vi "ParseSlaveRWw.vi"(1 "Node RWw":u16[][](array[numeric])) -> (0 "力觉力":sgl[](array[numeric]) format="%.2f")   [LabVIEW 2018]
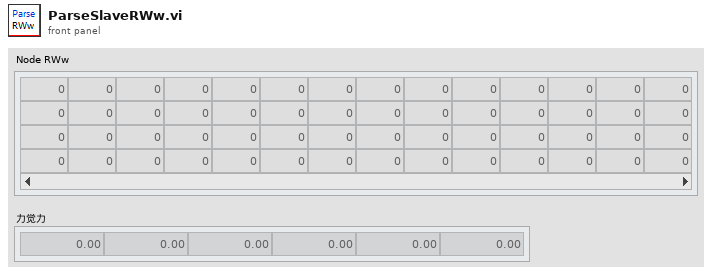
[diagram p1: front panel]
types:
  T1 = cluster{"1#当前泄漏量":sgl, "1#稳定泄漏量":sgl, "1#当前压力":sgl, "1#稳定压力":sgl, "1#风门闭电压":sgl, "1#风门开电压":sgl, "1#LED电流":sgl, "1#LED电压":sgl, "2#当前泄漏量":sgl, "2#稳定泄漏量":sgl, "2#当前压力":sgl, "2#稳定压力":sgl, "2#风门闭电压":sgl, "2#风门开电压":sgl, "2#LED电流":sgl, "2#LED电压":sgl, "3#当前泄漏量":sgl, "3#稳定泄漏量":sgl, "3#当前压力":sgl, "3#稳定压力":sgl, "3#风门闭电压":sgl, "3#风门开电压":sgl, "3#LED电流":sgl, "3#LED电压":sgl}
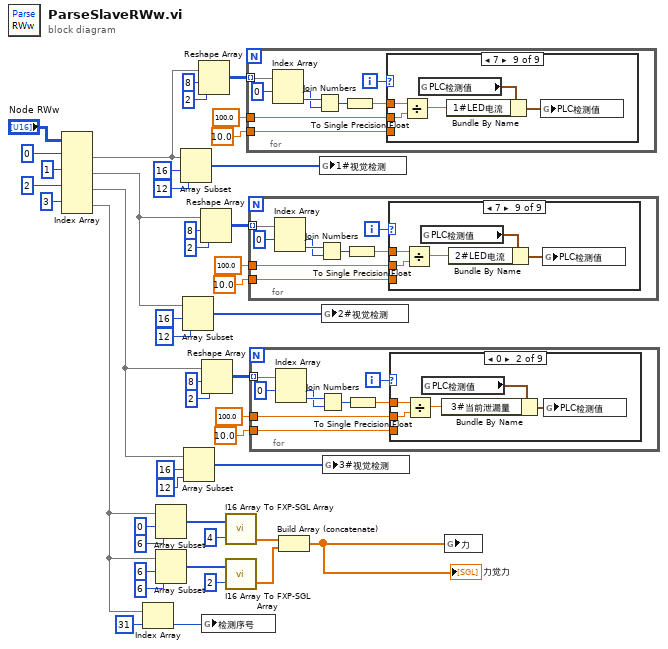
[diagram p0: block diagram]
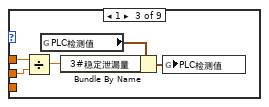
[diagram p3: hidden frame]
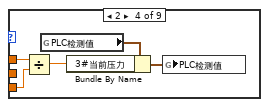
[diagram p4: hidden frame]
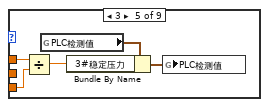
[diagram p5: hidden frame]
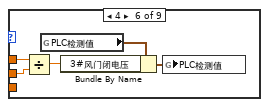
[diagram p6: hidden frame]
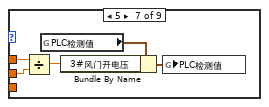
[diagram p7: hidden frame]
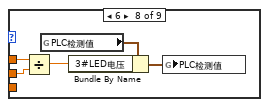
[diagram p8: hidden frame]
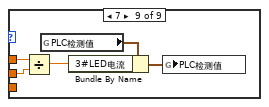
[diagram p9: hidden frame]
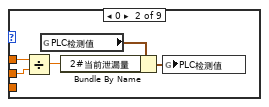
[diagram p11: hidden frame]
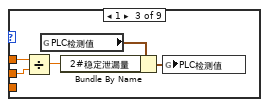
[diagram p12: hidden frame]
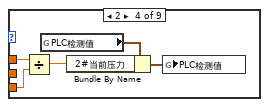
[diagram p13: hidden frame]
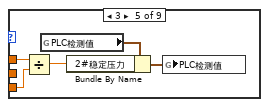
[diagram p14: hidden frame]
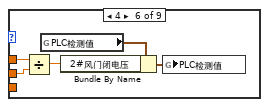
[diagram p15: hidden frame]
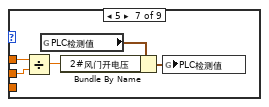
[diagram p16: hidden frame]
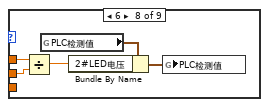
[diagram p17: hidden frame]
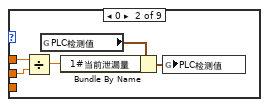
[diagram p19: hidden frame]
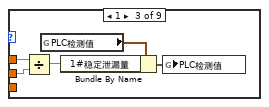
[diagram p20: hidden frame]
diagram:
  n1 = Index Array(array="Node RWw", index (row) #1=0 ("索引 (行)"), index (row) #2=1 ("索引 (行)"), index (row) #3=2 ("索引 (行)"), index (row) #4=3 ("索引 (行)")) -> (element #1=w39:u16[], element #2=w15:u16[], element #3=w6:u16[], element #4=w3:u16[])  [unwired: 4 in]
  n2 = Index Array(array=w3, index=31 ("索引")) -> (element=w1:u16)
  n3 = Array Subset(array=w3, index=0 ("索引"), length=6 ("长度")) -> (w33:u16[])
  n4 = Array Subset(array=w3, index=6 ("索引"), length=6 ("长度")) -> (w28:u16[])
  n5 = Array Subset(array=w39, index=16 ("索引"), length=12 ("长度")) -> (w36:u16[])
  n6 = Array Subset(array=w15, index=16 ("索引"), length=12 ("长度")) -> (w16:u16[])
  n7 = Array Subset(array=w6, index=16 ("索引"), length=12 ("长度")) -> (w7:u16[])
  n8 = Reshape Array(w39, 8 ("维数大小"), 2 ("维数大小")) -> (w42:u16[][])
  n9 = Reshape Array(w15, 8 ("维数大小"), 2 ("维数大小")) -> (w21:u16[][])
  n10 = Reshape Array(w6, 8 ("维数大小"), 2 ("维数大小")) -> (w12:u16[][])
  n11 = global write "全局 1.vi" "检测序号"(w1) -> ()
  n12 = call "I16 Array To FXP-SGL Array.vi"("小数位数"=4, "I16 Array"=w33) -> ("SGL Array"=w26:sgl[])  [unwired: 1 out]
  n13 = call "I16 Array To FXP-SGL Array.vi"("小数位数"=2, "I16 Array"=w28) -> ("SGL Array"=w25:sgl[])  [unwired: 1 out]
  n14 = for {
    tunnel: w42 -> [w55] mode=indexing
    tunnel: sgl 100.0 -> [w49]
    tunnel: sgl 10.0 -> [w48]
    i -> [w47]
    n15 = Index Array(array=w55, index #1=0 ("索引")) -> (element #1=w52:u16, element #2=w53:u16)  [unwired: 1 in]
    n16 = Join Numbers(hi=w53, lo=w52) -> ((hi.lo)=w51:u32)
    n17 = To Single Precision Float(number=w51) -> (single precision float=w50:sgl)
    n18 = case shown="7" w47 {
      tunnel: w50 -> [_ w60 w65 w70 w75 w80 w85 w90 w95]
      tunnel: w49 -> [_ w59 w64 _ _ w79 w84 w89 w91]
      tunnel: w48 -> [_ _ _ w66 w71 _ _ _ _]
      frame -1, Default {
      }
      frame 0 {
        n19 = Divide(x=w60, y=w59) -> (x/y=w58:sgl)
        n20 = global read "全局 1.vi" "PLC检测值"() -> (w56:T1)
        n21 = Bundle By Name(cluster=w56, "1#当前泄漏量"=w58) -> (w57:T1)
        n22 = global write "全局 1.vi" "PLC检测值"(w57) -> ()
      }
      frame 1 {
        n23 = Divide(x=w65, y=w64) -> (x/y=w63:sgl)
        n24 = global read "全局 1.vi" "PLC检测值"() -> (w61:T1)
        n25 = Bundle By Name(cluster=w61, "1#稳定泄漏量"=w63) -> (w62:T1)
        n26 = global write "全局 1.vi" "PLC检测值"(w62) -> ()
      }
      frame 2 {
        n27 = Divide(x=w70, y=w66) -> (x/y=w69:sgl)
        n28 = global read "全局 1.vi" "PLC检测值"() -> (w67:T1)
        n29 = Bundle By Name(cluster=w67, "1#当前压力"=w69) -> (w68:T1)
        n30 = global write "全局 1.vi" "PLC检测值"(w68) -> ()
      }
      frame 3 {
        n31 = Divide(x=w75, y=w71) -> (x/y=w74:sgl)
        n32 = global read "全局 1.vi" "PLC检测值"() -> (w72:T1)
        n33 = Bundle By Name(cluster=w72, "1#稳定压力"=w74) -> (w73:T1)
        n34 = global write "全局 1.vi" "PLC检测值"(w73) -> ()
      }
      frame 4 {
        n35 = Divide(x=w80, y=w79) -> (x/y=w78:sgl)
        n36 = global read "全局 1.vi" "PLC检测值"() -> (w76:T1)
        n37 = Bundle By Name(cluster=w76, "1#风门闭电压"=w78) -> (w77:T1)
        n38 = global write "全局 1.vi" "PLC检测值"(w77) -> ()
      }
      frame 5 {
        n39 = Divide(x=w85, y=w84) -> (x/y=w83:sgl)
        n40 = global read "全局 1.vi" "PLC检测值"() -> (w81:T1)
        n41 = Bundle By Name(cluster=w81, "1#风门开电压"=w83) -> (w82:T1)
        n42 = global write "全局 1.vi" "PLC检测值"(w82) -> ()
      }
      frame 6 {
        n43 = Divide(x=w90, y=w89) -> (x/y=w88:sgl)
        n44 = global read "全局 1.vi" "PLC检测值"() -> (w86:T1)
        n45 = Bundle By Name(cluster=w86, "1#LED电压"=w88) -> (w87:T1)
        n46 = global write "全局 1.vi" "PLC检测值"(w87) -> ()
      }
      frame 7 {
        n47 = Divide(x=w95, y=w91) -> (x/y=w94:sgl)
        n48 = global read "全局 1.vi" "PLC检测值"() -> (w92:T1)
        n49 = Bundle By Name(cluster=w92, "1#LED电流"=w94) -> (w93:T1)
        n50 = global write "全局 1.vi" "PLC检测值"(w93) -> ()
      }
    }
  }
  n51 = for {
    tunnel: w21 -> [w104] mode=indexing
    tunnel: sgl 100.0 -> [w98]
    tunnel: sgl 10.0 -> [w97]
    i -> [w96]
    n52 = Index Array(array=w104, index #1=0 ("索引")) -> (element #1=w101:u16, element #2=w102:u16)  [unwired: 1 in]
    n53 = Join Numbers(hi=w102, lo=w101) -> ((hi.lo)=w100:u32)
    n54 = To Single Precision Float(number=w100) -> (single precision float=w99:sgl)
    n55 = case shown="7" w96 {
      tunnel: w99 -> [_ w109 w114 w119 w124 w129 w134 w139 w144]
      tunnel: w98 -> [_ w108 w113 _ _ w128 w133 w138 w140]
      tunnel: w97 -> [_ _ _ w115 w120 _ _ _ _]
      frame -1, Default {
      }
      frame 0 {
        n56 = Divide(x=w109, y=w108) -> (x/y=w107:sgl)
        n57 = global read "全局 1.vi" "PLC检测值"() -> (w105:T1)
        n58 = Bundle By Name(cluster=w105, "2#当前泄漏量"=w107) -> (w106:T1)
        n59 = global write "全局 1.vi" "PLC检测值"(w106) -> ()
      }
      frame 1 {
        n60 = Divide(x=w114, y=w113) -> (x/y=w112:sgl)
        n61 = global read "全局 1.vi" "PLC检测值"() -> (w110:T1)
        n62 = Bundle By Name(cluster=w110, "2#稳定泄漏量"=w112) -> (w111:T1)
        n63 = global write "全局 1.vi" "PLC检测值"(w111) -> ()
      }
      frame 2 {
        n64 = Divide(x=w119, y=w115) -> (x/y=w118:sgl)
        n65 = global read "全局 1.vi" "PLC检测值"() -> (w116:T1)
        n66 = Bundle By Name(cluster=w116, "2#当前压力"=w118) -> (w117:T1)
        n67 = global write "全局 1.vi" "PLC检测值"(w117) -> ()
      }
      frame 3 {
        n68 = Divide(x=w124, y=w120) -> (x/y=w123:sgl)
        n69 = global read "全局 1.vi" "PLC检测值"() -> (w121:T1)
        n70 = Bundle By Name(cluster=w121, "2#稳定压力"=w123) -> (w122:T1)
        n71 = global write "全局 1.vi" "PLC检测值"(w122) -> ()
      }
      frame 4 {
        n72 = Divide(x=w129, y=w128) -> (x/y=w127:sgl)
        n73 = global read "全局 1.vi" "PLC检测值"() -> (w125:T1)
        n74 = Bundle By Name(cluster=w125, "2#风门闭电压"=w127) -> (w126:T1)
        n75 = global write "全局 1.vi" "PLC检测值"(w126) -> ()
      }
      frame 5 {
        n76 = Divide(x=w134, y=w133) -> (x/y=w132:sgl)
        n77 = global read "全局 1.vi" "PLC检测值"() -> (w130:T1)
        n78 = Bundle By Name(cluster=w130, "2#风门开电压"=w132) -> (w131:T1)
        n79 = global write "全局 1.vi" "PLC检测值"(w131) -> ()
      }
      frame 6 {
        n80 = Divide(x=w139, y=w138) -> (x/y=w137:sgl)
        n81 = global read "全局 1.vi" "PLC检测值"() -> (w135:T1)
        n82 = Bundle By Name(cluster=w135, "2#LED电压"=w137) -> (w136:T1)
        n83 = global write "全局 1.vi" "PLC检测值"(w136) -> ()
      }
      frame 7 {
        n84 = Divide(x=w144, y=w140) -> (x/y=w143:sgl)
        n85 = global read "全局 1.vi" "PLC检测值"() -> (w141:T1)
        n86 = Bundle By Name(cluster=w141, "2#LED电流"=w143) -> (w142:T1)
        n87 = global write "全局 1.vi" "PLC检测值"(w142) -> ()
      }
    }
  }
  n88 = for {
    tunnel: w12 -> [w153] mode=indexing
    tunnel: sgl 100.0 -> [w147]
    tunnel: sgl 10.0 -> [w146]
    i -> [w145]
    n89 = Index Array(array=w153, index #1=0 ("索引")) -> (element #1=w150:u16, element #2=w151:u16)  [unwired: 1 in]
    n90 = Join Numbers(hi=w151, lo=w150) -> ((hi.lo)=w149:u32)
    n91 = To Single Precision Float(number=w149) -> (single precision float=w148:sgl)
    n92 = case shown="0" w145 {
      tunnel: w148 -> [_ w158 w163 w168 w173 w178 w183 w188 w193]
      tunnel: w147 -> [_ w157 w162 _ _ w177 w182 w187 w189]
      tunnel: w146 -> [_ _ _ w164 w169 _ _ _ _]
      frame -1, Default {
      }
      frame 0 {
        n93 = Divide(x=w158, y=w157) -> (x/y=w156:sgl)
        n94 = global read "全局 1.vi" "PLC检测值"() -> (w154:T1)
        n95 = Bundle By Name(cluster=w154, "3#当前泄漏量"=w156) -> (w155:T1)
        n96 = global write "全局 1.vi" "PLC检测值"(w155) -> ()
      }
      frame 1 {
        n97 = Divide(x=w163, y=w162) -> (x/y=w161:sgl)
        n98 = global read "全局 1.vi" "PLC检测值"() -> (w159:T1)
        n99 = Bundle By Name(cluster=w159, "3#稳定泄漏量"=w161) -> (w160:T1)
        n100 = global write "全局 1.vi" "PLC检测值"(w160) -> ()
      }
      frame 2 {
        n101 = Divide(x=w168, y=w164) -> (x/y=w167:sgl)
        n102 = global read "全局 1.vi" "PLC检测值"() -> (w165:T1)
        n103 = Bundle By Name(cluster=w165, "3#当前压力"=w167) -> (w166:T1)
        n104 = global write "全局 1.vi" "PLC检测值"(w166) -> ()
      }
      frame 3 {
        n105 = Divide(x=w173, y=w169) -> (x/y=w172:sgl)
        n106 = global read "全局 1.vi" "PLC检测值"() -> (w170:T1)
        n107 = Bundle By Name(cluster=w170, "3#稳定压力"=w172) -> (w171:T1)
        n108 = global write "全局 1.vi" "PLC检测值"(w171) -> ()
      }
      frame 4 {
        n109 = Divide(x=w178, y=w177) -> (x/y=w176:sgl)
        n110 = global read "全局 1.vi" "PLC检测值"() -> (w174:T1)
        n111 = Bundle By Name(cluster=w174, "3#风门闭电压"=w176) -> (w175:T1)
        n112 = global write "全局 1.vi" "PLC检测值"(w175) -> ()
      }
      frame 5 {
        n113 = Divide(x=w183, y=w182) -> (x/y=w181:sgl)
        n114 = global read "全局 1.vi" "PLC检测值"() -> (w179:T1)
        n115 = Bundle By Name(cluster=w179, "3#风门开电压"=w181) -> (w180:T1)
        n116 = global write "全局 1.vi" "PLC检测值"(w180) -> ()
      }
      frame 6 {
        n117 = Divide(x=w188, y=w187) -> (x/y=w186:sgl)
        n118 = global read "全局 1.vi" "PLC检测值"() -> (w184:T1)
        n119 = Bundle By Name(cluster=w184, "3#LED电压"=w186) -> (w185:T1)
        n120 = global write "全局 1.vi" "PLC检测值"(w185) -> ()
      }
      frame 7 {
        n121 = Divide(x=w193, y=w189) -> (x/y=w192:sgl)
        n122 = global read "全局 1.vi" "PLC检测值"() -> (w190:T1)
        n123 = Bundle By Name(cluster=w190, "3#LED电流"=w192) -> (w191:T1)
        n124 = global write "全局 1.vi" "PLC检测值"(w191) -> ()
      }
    }
  }
  n125 = Build Array (concatenate)(w26, w25) -> (w24:sgl[])
  "力觉力" <- w24
  n126 = global write "全局 1.vi" "1#视觉检测"(w36) -> ()
  n127 = global write "全局 1.vi" "2#视觉检测"(w16) -> ()
  n128 = global write "全局 1.vi" "3#视觉检测"(w7) -> ()
  n129 = global write "全局 1.vi" "力"(w24) -> ()
